vi "Write Setpoint.vi"(8 "error in (no error)":errorcluster, 10 "Setpoint":dbl=1.0, 11 "Percent Difference in":refnum<class "Percent Difference.lvclass">) -> (0 "error out":errorcluster, 3 "Percent Difference out":refnum<class "Percent Difference.lvclass">)   [LabVIEW 2021, in "Percent Difference.lvclass"]
uses:
  Percent Difference.lvclass
  Percent Difference.lvclass/Percent Difference.ctl
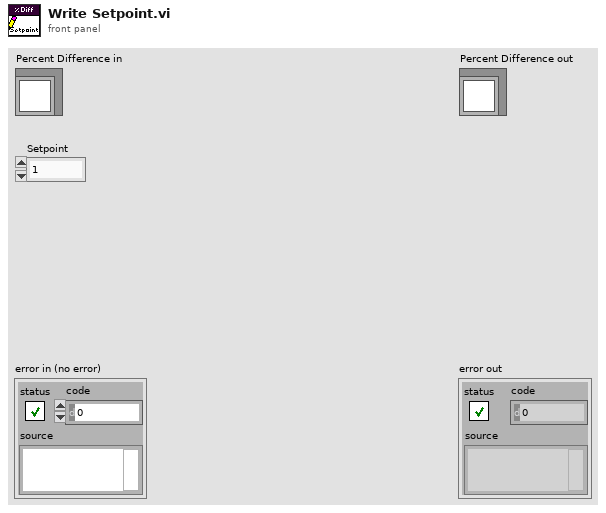
[diagram p1: front panel]
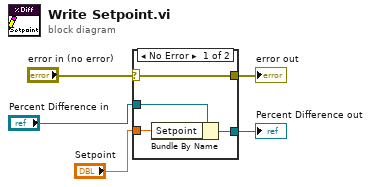
[diagram p0: block diagram]
diagram:
  n1 = case shown="No Error" "error in (no error)" {
    selector: "error in (no error)" -> [w9 w10]
    tunnel: [w9 w10] -> w4
    tunnel: [w7 w11] -> w2
    tunnel: "Percent Difference in" -> [w8 w11]
    tunnel: "Setpoint" -> [w6 _]
    frame No Error {
      n2 = Bundle By Name(cluster=w8, "Setpoint"=w6) -> (w7:refnum<class "Percent Difference.lvclass">)
    }
    frame Error {
    }
  }
  "error out" <- w4
  "Percent Difference out" <- w2
